vi "9214_Initialize.vi"(7 "Module Model":T1=enum."NI 9205", 8 "error in (no error)":errorcluster, 9 "Slot Settings":T2) -> (0 "error out":errorcluster, 3 "9214 out":refnum<class "9214.lvclass">)   [LabVIEW 2017, in "Modules.lvlib" / "9214.lvclass"]
uses:
  9214.lvclass
  RSI Module/Slot Settings.ctl
  C:/Users/dbuck/Documents/GitHub/Scan-Engine-Custom-Device-Classes/Source/9213/9213.lvclass
  C:/Users/dbuck/Documents/GitHub/Scan-Engine-Custom-Device-Classes/Source/RSI Module/RSI Module.lvclass
  RSI Module/Module Models.ctl
  9214.lvclass/9214.ctl
  9213/9213.lvclass
  RSI Module/RSI Module.lvclass
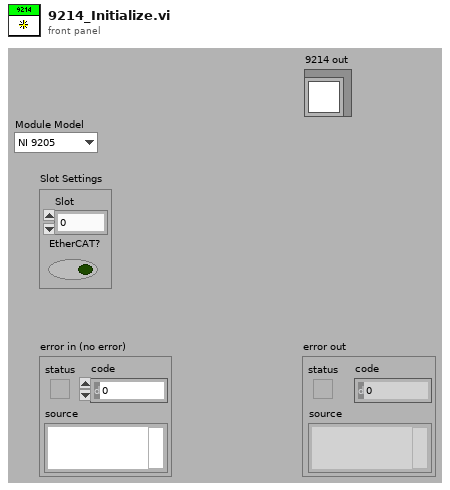
[diagram p1: front panel]
types:
  T1 = typedef "Modules.lvlib/RSI Module.lvclass/Module Models.ctl" = enum16{"Empty", "NI 9201", "NI 9203", "NI 9205", "NI 9206", "NI 9207", "NI 9208", "NI 9211", "NI 9212", "NI 9213", "NI 9214", "NI 9215", "NI 9217", "NI 9219", "NI 9220", "NI 9221", "NI 9222", "NI 9223", "NI 9225", "NI 9227", "NI 9229", "NI 9233", "NI 9234", "NI 9235", "NI 9236", "NI 9237", "NI 9239", "NI 9242", "NI 9244", "NI 9263", "NI 9264", "NI 9265", "NI 9269", "NI 9375", "NI 9401", "NI 9402", "NI 9403", "NI 9411", "NI 9421", "NI 9422", "NI 9423", "NI 9425", "NI 9426", "NI 9435", "NI 9437", "NI 9472", "NI 9474", "NI 9475", "NI 9476", "NI 9477", "NI 9478", "NI 9481", "NI 9482", "NI 9485"}
  T2 = typedef "Modules.lvlib/RSI Module.lvclass/Slot Settings.ctl" = cluster{"Slot":u32, "EtherCAT?":bool}
  T3 = typedef "Modules.lvlib/RSI Module.lvclass/Channels.ctl" = cluster{"# Input Channels":i32, "# Output Channels":i32, "Channel Type":T4, "Units":string}
  T4 = typedef "Modules.lvlib/RSI Module.lvclass/Channel Type.ctl" = enum16{"Analog", "Digital"}
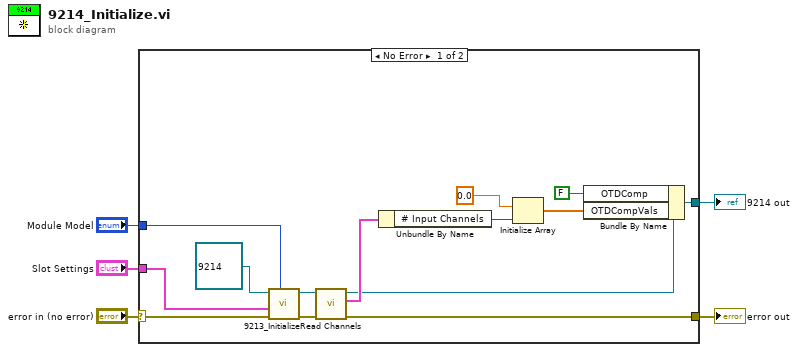
[diagram p0: block diagram]
diagram:
  n1 = case shown="No Error" "error in (no error)" {
    selector: "error in (no error)" -> [w19 w20]
    tunnel: [w9 w20] -> w4
    tunnel: [w18 _] -> w3
    tunnel: "Slot Settings" -> [w15 _]
    tunnel: "Module Model" -> [w14 _]
    frame No Error {
      n2 = call "9213_Initialize.vi"("Module Model"=w14, "error in (no error)"=w19, "Slot Settings"=w15, "9213 in"=refnum<class "9214.lvclass"> refnum ("Modules.lvlib:9214.lvclass")) -> ("error out"=w12:errorcluster, "9213 out"=w13:refnum<class "9214.lvclass">)  [unwired: 6 in]
      n3 = call "Read Channels.vi"("error in (no error)"=w12, "RSI Module in"=w13) -> ("error out"=w9:errorcluster, "Channels"=w11:T3, "RSI Module out"=w10:refnum<class "9214.lvclass">)  [unwired: 7 in]
      n4 = Unbundle By Name(w11) -> ("# Input Channels"=w8:i32)
      n5 = Initialize Array(0.0, w8) -> (w6:dbl[])
      n6 = Bundle By Name(cluster=w10, "OTDComp"=FALSE, "OTDCompVals"=w6) -> (w18:refnum<class "9214.lvclass">)
    }
    frame Error {
    }
  }
  "error out" <- w4
  "9214 out" <- w3
